vi "buildStartCycle.vi"(8 "error in (no error)":errorcluster, 11 "ICommandBuilder in":refnum<class "ICommandBuilder.lvclass">) -> (0 "error out":errorcluster, 3 "ICommandBuilder out":refnum<class "ICommandBuilder.lvclass">)   [LabVIEW 2023, in "ICommandBuilder.lvclass"]
uses:
  ICommandBuilder.lvclass
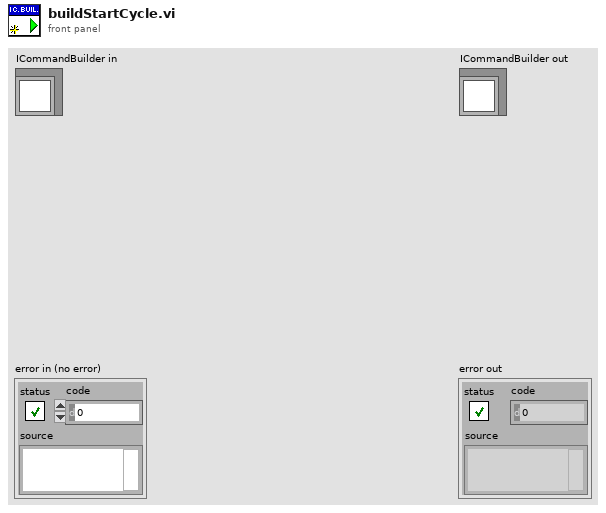
[diagram p1: front panel]
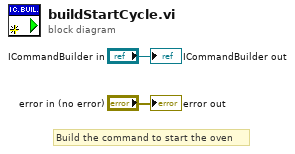
[diagram p0: block diagram]
diagram:
  # "Build the command to start the oven"
  "error out" <- "error in (no error)"
  "ICommandBuilder out" <- "ICommandBuilder in"
